vi "Linear Fit Coefficients (Bisquare).vi"(0 "Y":dbl[](array[numeric]) format="%#.6g", 5 "X":dbl[](array[numeric]) format="%#.6g", 7 "Weight":dbl[](array[numeric]) format="%#.6g", 9 "tol":dbl=0.0001) -> (4 "slope":dbl format="%#.6g", 6 "intercept":dbl format="%#.6g", 15 "error":i32)   [LabVIEW 2020, in "NI_AALPro.lvlib"]
uses:
  <vilib>/Analysis/NI_AALPro.lvlib
  <resource>/lvanlys.dll
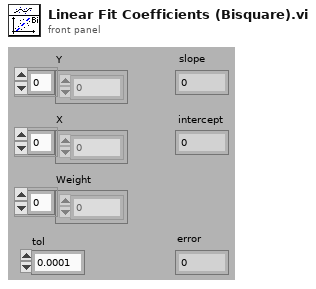
[diagram p1: front panel]
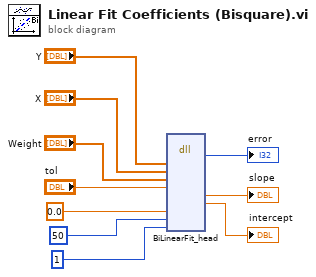
[diagram p0: block diagram]
diagram:
  n1 = dll-call lib="e:/builds/penguin/labview/branches/2020/dev/dist/resource/lvanlys.*" fn="BiLinearFit_head"("yH"="Y", "xH"="X", "weight"="Weight", "tol"="tol", "meanErr"=0.0 ("absTol"), "maxIter"=50, "isCoef"=1) -> (→"error":i32, "slope"=→"slope":dbl, "intercept"=→"intercept":dbl)  [unwired: 12 in, 2 out]
